vi "Read Signal List.vi"(8 "error in":errorcluster, 11 "file path (use dialog)":path) -> (0 "error out":errorcluster, 3 "Names":T1)   [LabVIEW 2020]
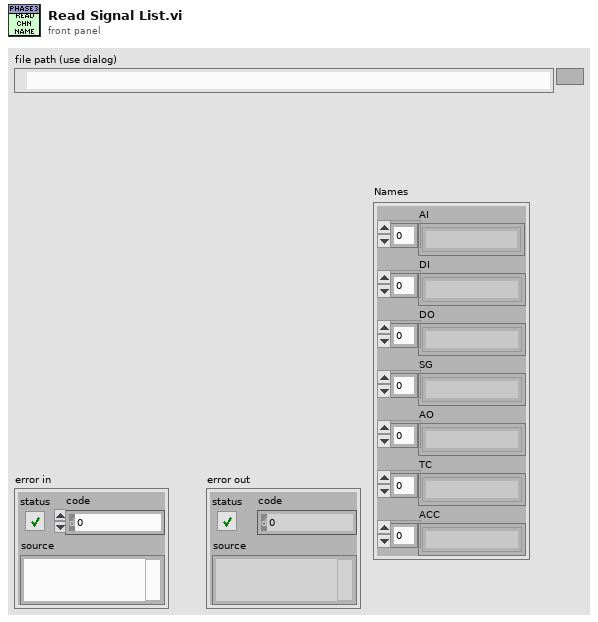
[diagram p1: front panel]
types:
  T1 = cluster{"AI":string[], "DI":string[], "DO":string[], "SG":string[], "AO":string[], "TC":string[], "ACC":string[]}
  T2 = enum16{"open", "replace", "create", "open or create", "replace or create", "replace or create with confirmation"}
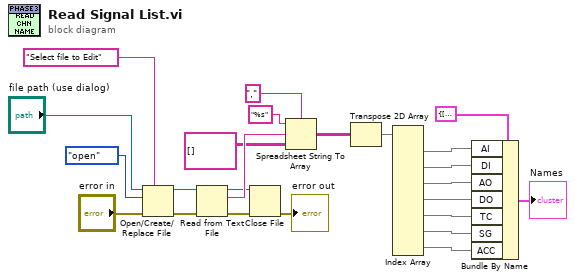
[diagram p0: block diagram]
diagram:
  n1 = Open/Create/Replace File(file path (use dialog)="file path (use dialog)", error in="error in", prompt="Select file to Edit", operation (0:open)=T2."open") -> (refnum out=w21:refnum<file>, error out=w20:errorcluster)  [unwired: 2 in, 1 out]
  n2 = Read from Text File(file (use dialog)=w21, error in=w20) -> (refnum out=w23:refnum<file>, text=w24:string, error out=w22:errorcluster)  [unwired: 2 in, 1 out]
  n3 = Close File(refnum=w23, error in=w22) -> (error out=→"error out":errorcluster)  [unwired: 1 out]
  n4 = Spreadsheet String To Array(delimiter (Tab)=",", format string="%s", spreadsheet string=w24, array type (2D Dbl)=string[][] [] ("Table Control")) -> (array=w11:string[][])
  n5 = Transpose 2D Array(2D array=w11) -> (transposed array=w8:string[][])
  n6 = Index Array(array=w8) -> (element #1=w7:string[], element #2=w6:string[], element #3=w5:string[], element #4=w4:string[], element #5=w3:string[], element #6=w2:string[], element #7=w1:string[])  [unwired: 14 in]
  n7 = Bundle By Name(cluster=T1 {"AI"=[], "DI"=[], "DO"=[], "SG"=[], "AO"=[], "TC"=[], "ACC"=[]} ("Cluster"), "AI"=w7, "DI"=w6, "AO"=w5, "DO"=w4, "TC"=w3, "SG"=w2, "ACC"=w1) -> (→"Names":T1)
